vi "Initialize Tag.vi"(6 "Units":string, 7 "Keyword":string, 8 "error in (no error)":errorcluster, 9 "Data Type":string(combo)="Double", 10 "Tag Name":string, 11 "Logger in.lvclass":refnum<class "Logger.lvclass">) -> (0 "error out":errorcluster, 3 "Logger out.lvclass":refnum<class "Logger.lvclass">)   [LabVIEW 2019, in "Logger.lvclass"]
uses:
  Logger.lvclass
  Logger.lvclass/Logger.ctl
  <vilib>/Skyline/Tag/Shared/typedefs/TagProperty.ctl
  <vilib>/Skyline/Tag/Shared/typedefs/DataType.ctl
  <vilib>/Skyline/Tag/Wrapper/Wrapper AMQP_class/Open Tag AMQP.vi
  <vilib>/Skyline/Tag/Wrapper/Wrapper_class/NI Skyline Tag.lvclass
  <vilib>/Skyline/Tag/Shared/NI Skyline Tag.lvlib
  <vilib>/Skyline/Tag/Wrapper/Wrapper AMQP_class/NI Skyline Tag AMQP.lvclass
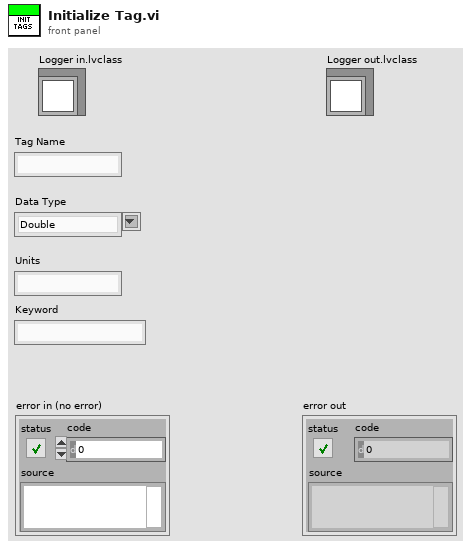
[diagram p1: front panel]
types:
  T1 = typedef "NI Skyline Tag.lvlib/DataType.ctl" = enum32{"Double", "I32", "String", "Boolean", "U64", "Timestamp"}
  T2 = typedef "NI Skyline Tag.lvlib/TagProperty.ctl" = cluster{"key":string, "value":string}
  T3 = cluster{"Tag Units":string, "Tag Path":string, "Tag Reference":refnum<class "NI Skyline Tag.lvclass">}[]
  T4 = cluster{"Tag Units":string, "Tag Path":string, "Tag Reference":refnum<class "NI Skyline Tag.lvclass">}
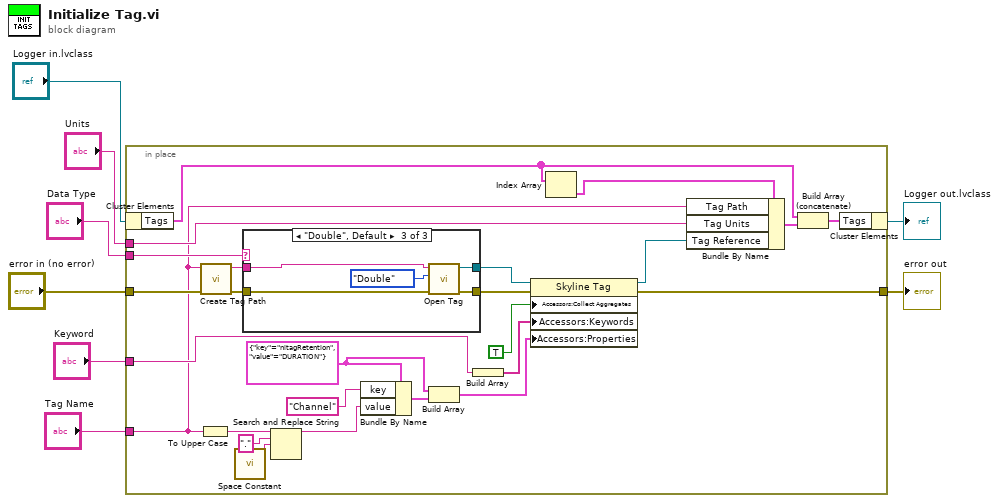
[diagram p0: block diagram]
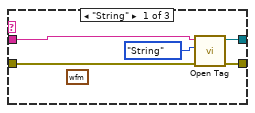
[diagram p2: hidden frame]
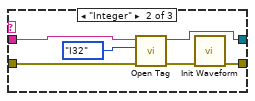
[diagram p3: hidden frame]
diagram:
  n1 = in-place {
    in-place-border: [w26] -> w8
    in-place-border: "Tag Name" -> [w13]
    in-place-border: "Data Type" -> [w33]
    in-place-border: "Units" -> [w32]
    in-place-border: "error in (no error)" -> [w21]
    in-place-border: "Keyword" -> [w23]
    w18 = T2 {"key"="nitagRetention", "value"="DURATION"} ("Property")
    n2 = in-place-cluster #1("Logger in.lvclass") -> ("Tags"=w10:T3)
    n3 = To Upper Case(1:w13) -> (0:w16:string)
    n4 = call "Create Tag Path.vi"("error in (no error)"=w21, "tag name"=w13) -> ("error out"=w20:errorcluster, "path"=w31:string)  [unwired: 8 in]
    n5 = call <vilib>:"Space Constant.vi"() -> ("String"=w14:string)
    n6 = case shown="\"Double\", Default" w33 {
      tunnel: [w36 w44 w45] -> w27
      tunnel: [w37 w40 w46] -> w25
      tunnel: w31 -> [w35 w42 w47]
      tunnel: w20 -> [w38 w43 w49]
      frame "String" {
        (unwired) waveform(dbl) {"t0"=timestamp(0 s since 1904-01-01), "dt"=1.0, "Y"=[]} ("waveform")
        n7 = call-poly <vilib>:"Open Tag.vi"("error in (no error)"=w38, "data type"=DataType."String" ("Data Type"), "path"=w35) -> ("error out"=w36:errorcluster, "tag"=w37:refnum<class "NI Skyline Tag.lvclass">)  [unwired: 7 in]
      }
      frame "Integer" {
        n8 = call-poly <vilib>:"Open Tag.vi"("error in (no error)"=w43, "data type"=DataType."I32", "path"=w42) -> ("error out"=w41:errorcluster, "tag"=w40:refnum<class "NI Skyline Tag.lvclass">)  [unwired: 7 in]
        n9 = call "Init Waveform.vi"("error in (no error)"=w41) -> ("error out"=w44:errorcluster)  [unwired: 9 in, 1 out]
      }
      frame "Double", Default {
        n10 = call-poly <vilib>:"Open Tag.vi"("error in (no error)"=w49, "data type"=DataType."Double" ("Data Type"), "path"=w47) -> ("error out"=w45:errorcluster, "tag"=w46:refnum<class "NI Skyline Tag.lvclass">)  [unwired: 7 in]
      }
    }
    n11 = Search and Replace String(input string=w16, search string=".", replace string=w14) -> (result string=w11:string)  [unwired: 5 in, 3 out]
    n12 = Bundle By Name(cluster=w18, "key"="Channel", "value"=w11) -> (w17:T2)
    n13 = Build Array(w18, w17) -> (w19:T2[])
    n14 = Build Array(w23) -> (w22:string[])
    n15 = property class="Skyline Tag"(reference=w25, error in=w27, "Accessors:Collect Aggregates"=TRUE ("Collect Aggregates"), "Accessors:Keywords"=w22, "Accessors:Properties"=w19) -> (reference out=w24:refnum<class "NI Skyline Tag.lvclass">, error out=w26:errorcluster)
    n16 = Index Array(array=w10) -> (element=w9:T4)  [unwired: 1 in]
    n17 = Bundle By Name(cluster=w9, "Tag Path"=w13, "Tag Units"=w32, "Tag Reference"=w24) -> (w29:T4)
    n18 = Build Array (concatenate)(w10, w29) -> (w30:T3)
    n19 = in-place-cluster #1("Tags"=w30) -> (→"Logger out.lvclass":refnum<class "Logger.lvclass">)
  }
  "error out" <- w8
